vi "Factory.vi"(8 "error in (no error)":errorcluster, 11 "Protocol Interface in":refnum<class "Protocol Interface.lvclass">) -> (0 "error out":errorcluster, 3 "Protocol Interface out":refnum<class "Protocol Interface.lvclass">)   [LabVIEW 2018, in "Protocol Interface.lvlib" / "Protocol Interface.lvclass"]
uses:
  Protocol Interface.lvclass
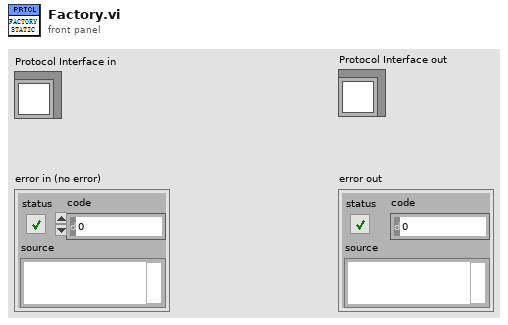
[diagram p1: front panel]
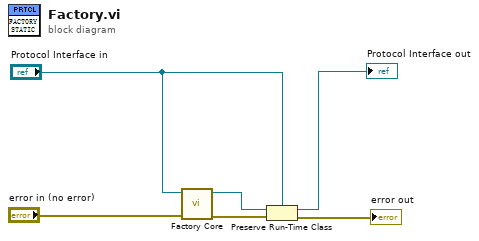
[diagram p0: block diagram]
diagram:
  n1 = call-dynamic "Factory Core.vi"("error in (no error)"="error in (no error)", "Protocol Interface in"="Protocol Interface in") -> ("error out"=w5:errorcluster, "Protocol Interface out"=w4:refnum<class "Protocol Interface.lvclass">)  [unwired: 8 in]
  n2 = Preserve Run-Time Class(object in=w4, error in=w5, 2:"Protocol Interface in") -> (object out=→"Protocol Interface out":refnum<class "Protocol Interface.lvclass">, error out=→"error out":errorcluster)
